vi "Throw JSON Error - Invalid Type Error.vi"(8 "error in (no error)":errorcluster, 9 "additional info":string, 11 "Valid Types":string[](array[string])) -> (0 "error out":errorcluster)   [LabVIEW 2014, in "i3-json.lvlib"]
uses:
  i3-json.lvlib
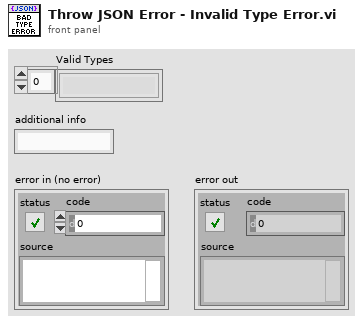
[diagram p1: front panel]
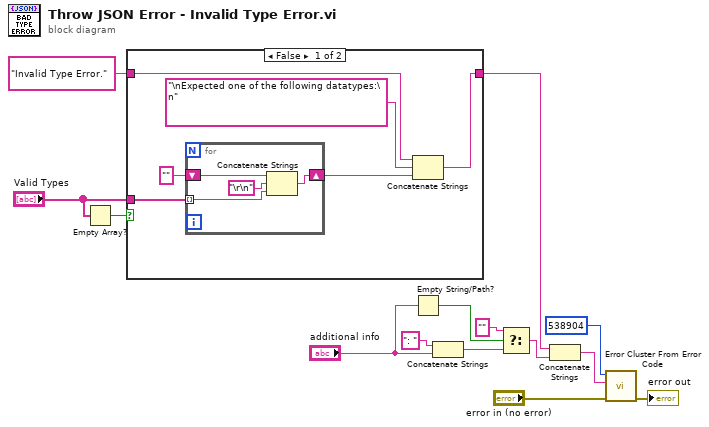
[diagram p0: block diagram]
diagram:
  n1 = Empty Array?(array="Valid Types") -> (empty?=w10:bool)
  n2 = case shown="False" w10 {
    tunnel: [w15 w25] -> w2
    tunnel: "Valid Types" -> [w19 _]
    tunnel: "Invalid Type Error." ("error message (\"\")") -> [w18 w25]
    frame False {
      n3 = for {
        shift-right: [w23] -> w16
        shift-left: "" -> [w21]
        tunnel: w19 -> [w22] mode=indexing
        n4 = Concatenate Strings(w21, "\r\n", w22) -> (w23:string)
      }
      n5 = Concatenate Strings(w18, "\nExpected one of the following datatypes:\n" ("string"), w16) -> (w15:string)
    }
    frame True {
    }
  }
  n6 = Empty String/Path?(string/path="additional info") -> (empty?=w8:bool)
  n7 = Concatenate Strings(": " ("string"), "additional info") -> (w3:string)
  n8 = Select(t="" ("datatype"), s=w8, f=w3) -> (s? t:f=w6:string)
  n9 = Concatenate Strings(w2, w6) -> (w1:string)
  n10 = call <vilib>:"Error Cluster From Error Code.vi"("error in (no error)"="error in (no error)", "error message (\"\")"=w1, "error code (0)"=538904) -> ("error out"=→"error out":errorcluster)  [unwired: 6 in]
